vi "serving  (SubVI).vi"(0 "1":bool, 4 "BR":bool, 5 "2":bool, 6 "BM":bool, 7 "3":bool, 8 "BL":bool, 10 "CR":bool, 11 "TL":bool, 12 "TM":bool, 13 "TR":bool, 14 "CL":bool, 15 "CM":bool) -> (2 "appended array":dbl[](array[numeric]))   [LabVIEW 2009]
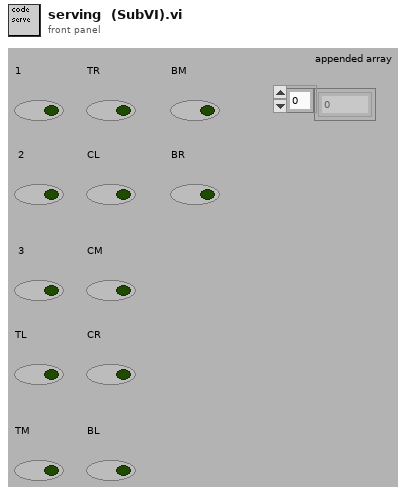
[diagram p1: front panel]
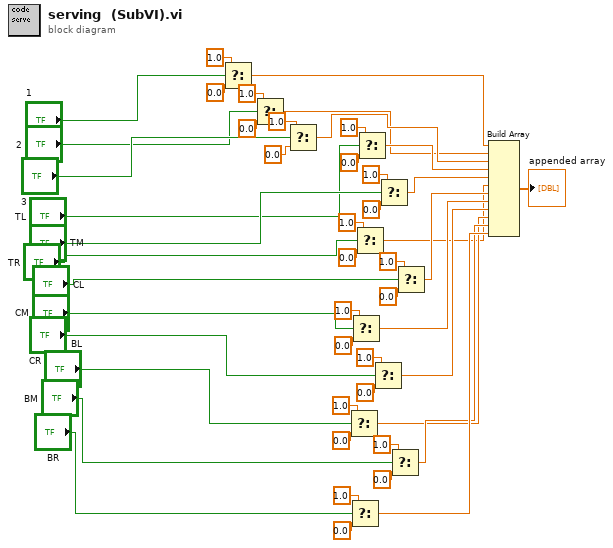
[diagram p0: block diagram]
diagram:
  n1 = Select(t=1.0, s="1", f=0.0) -> (s? t:f=w37:dbl)
  n2 = Select(t=1.0, s="2", f=0.0) -> (s? t:f=w38:dbl)
  n3 = Select(t=1.0, s="3", f=0.0) -> (s? t:f=w39:dbl)
  n4 = Select(t=1.0, s="BL", f=0.0) -> (s? t:f=w46:dbl)
  n5 = Select(t=1.0, s="BR", f=0.0) -> (s? t:f=w48:dbl)
  n6 = Select(t=1.0, s="CM", f=0.0) -> (s? t:f=w44:dbl)
  n7 = Select(t=1.0, s="TR", f=0.0) -> (s? t:f=w42:dbl)
  n8 = Select(t=1.0, s="TL", f=0.0) -> (s? t:f=w40:dbl)
  n9 = Select(t=1.0, s="CR", f=0.0) -> (s? t:f=w45:dbl)
  n10 = Select(t=1.0, s="TM", f=0.0) -> (s? t:f=w41:dbl)
  n11 = Select(t=1.0, s="BM", f=0.0) -> (s? t:f=w47:dbl)
  n12 = Select(t=1.0, s="CL", f=0.0) -> (s? t:f=w43:dbl)
  n13 = Build Array(w37, w38, w39, w40, w41, w42, w43, w44, w45, w46, w47, w48) -> (→"appended array":dbl[])
